vi "graphDyn.vi"() -> ()   [LabVIEW 2018]
panel:
  in  "Listbox":i32(listbox)
  out "Array 2":string[](array[string])
  out "Legend:Number of Rows":u32
  out "Waveform Graph":dbl[](graph)
  in  "nb SHT":i32
  in  "Stop":bool
  out "Array":cluster{"Waveform Graph":dbl[][]}[](array[cluster]) caption="0"
  in  "nb Box":i32
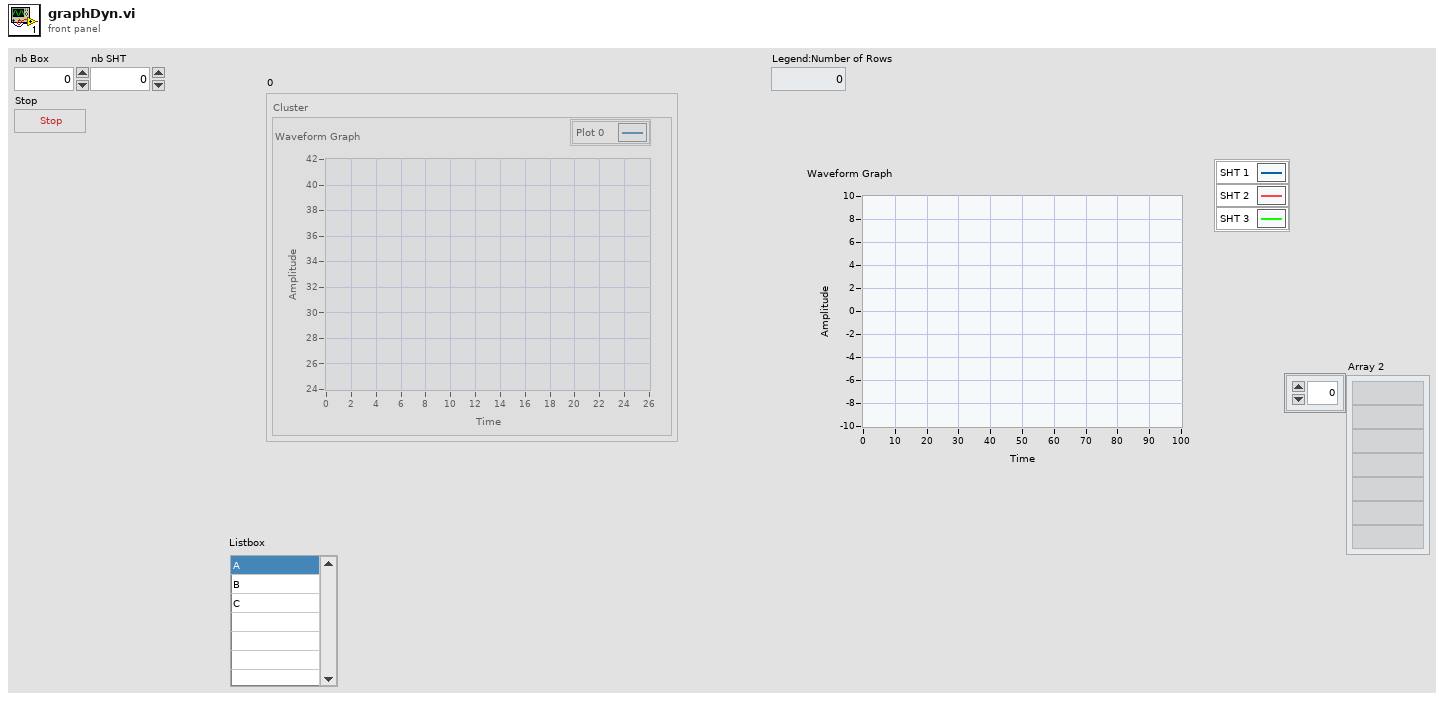
[diagram p1: front panel]
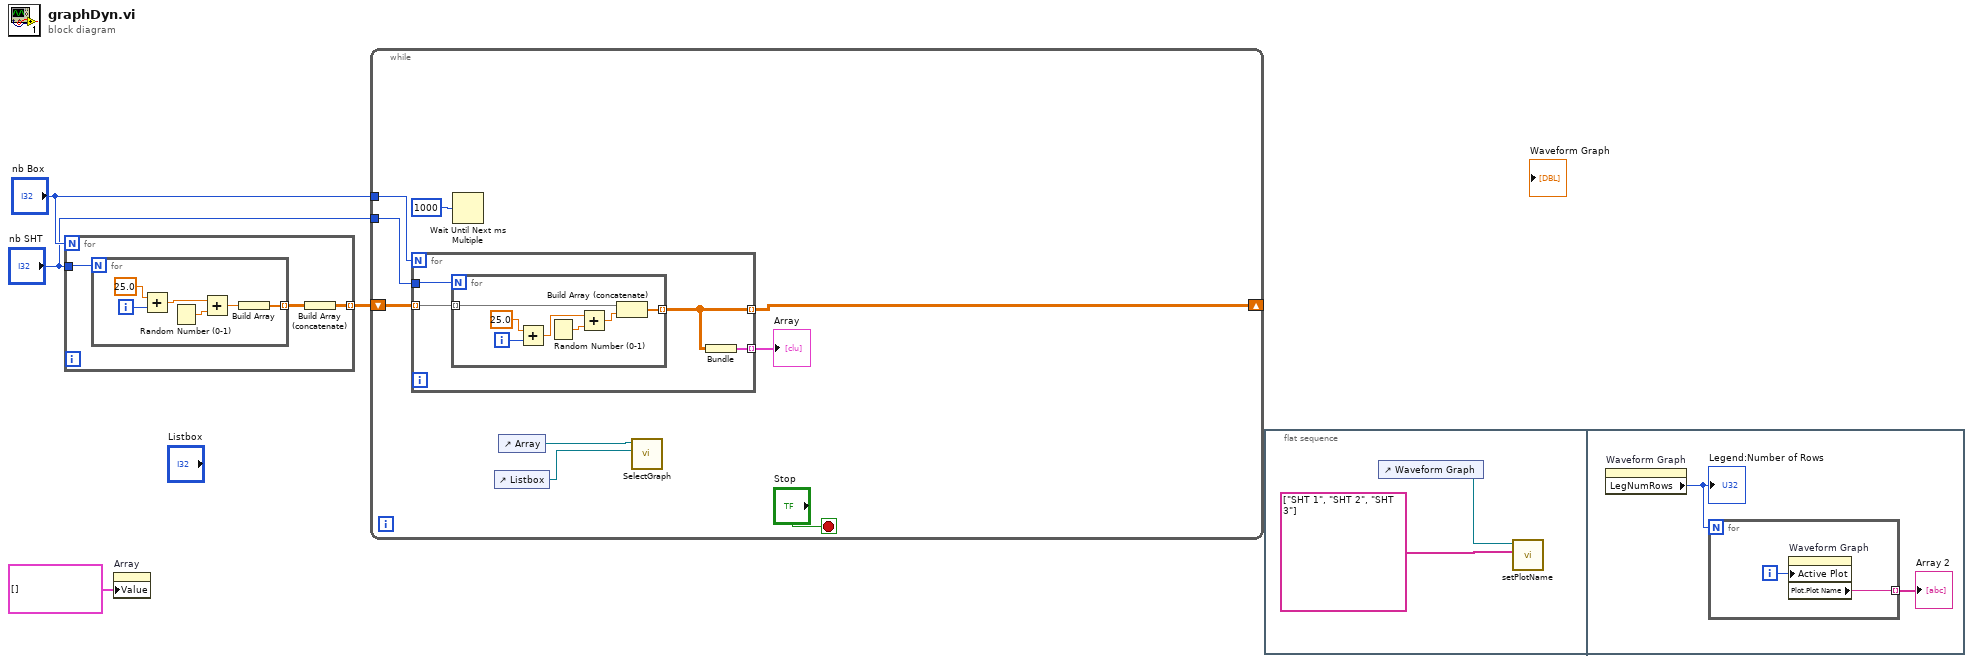
[diagram p0: block diagram]
diagram:
  n1 = for {
    N: "nb Box" -> [_]
    tunnel: "nb SHT" -> [w7]
    tunnel: [w5] -> w3 mode=indexing
    n2 = for {
      N: w7 -> [_]
      tunnel: [w13] -> w6 mode=indexing
      i -> [w11]
      n3 = Add(x=25.0, y=w11) -> (x+y=w10:dbl)
      n4 = Random Number (0-1)() -> (number: 0 to 1=w9:dbl)
      n5 = Add(x=w10, y=w9) -> (x+y=w8:dbl)
      n6 = Build Array(w8) -> (w13:dbl[])
    }
    n7 = Build Array (concatenate)(w6) -> (w5:dbl[][])
  }
  n8 = property on="Array" class="Arr (strict)"("Value"=cluster{"Waveform Graph":dbl[][]}[] [] ("Array")) -> ()  [unwired: 2 in, 2 out]
  n9 = while {
    shift-right: [w17] -> _
    shift-left: w3 -> [w21]
    tunnel: "nb Box" -> [w19]
    tunnel: "nb SHT" -> [w18]
    stop <- "Stop" stop-if-true
    n10 = for {
      N: w19 -> [_]
      tunnel: w21 -> [w24] mode=indexing
      tunnel: [w26] -> w16 mode=indexing
      tunnel: w18 -> [w25]
      tunnel: [w23] -> w17 mode=indexing
      n11 = for {
        N: w25 -> [_]
        tunnel: w24 -> [w33] mode=indexing
        tunnel: [w32] -> w23 mode=indexing
        i -> [w28]
        n12 = Add(x=25.0, y=w28) -> (x+y=w30:dbl)
        n13 = Random Number (0-1)() -> (number: 0 to 1=w31:dbl)
        n14 = Add(x=w30, y=w31) -> (x+y=w27:dbl)
        n15 = Build Array (concatenate)(w33, w27) -> (w32:dbl[])
      }
      n16 = Bundle(w23) -> (w26:cluster{dbl[][]})  [unwired: 1 in]
    }
    "Array" <- w16
    n17 = Wait Until Next ms Multiple(millisecond multiple=u32 1000) -> ()  [unwired: 1 out]
    n18 = control-ref of="Listbox"() -> (w14:refnum<vi>)
    n19 = control-ref of="Array"() -> (w15:refnum<vi>)
    n20 = call "SelectGraph.vi"("ListBox in"=w14, "Array in"=w15) -> ()  [unwired: 10 in]
  }
  n21 = flat-sequence {
    frame #0 {
      n22 = control-ref of="Waveform Graph"() -> (w34:refnum<vi>)
      n23 = call "setPlotName.vi"("Array 3"=string[] ["SHT 1", "SHT 2", "SHT 3"], "WaveformGraph in"=w34) -> ()  [unwired: 10 in]
    }
    frame #1 {
      n24 = property on="Waveform Graph" class="WFGraph (strict)"() -> ("LegNumRows"=w36:u32)  [unwired: 2 in, 2 out]
      "Legend:Number of Rows" <- w36
      n25 = for {
        N: w36 -> [_]
        tunnel: [w38] -> w37 mode=indexing
        i -> [w39]
        n26 = property on="Waveform Graph" class="WFGraph (strict)"("Active Plot"=w39) -> ("Plot.Plot Name"=w38:string)  [unwired: 2 in, 2 out]
      }
      "Array 2" <- w37
    }
  }
